vi "FindOutputLine.vi"(8 "error in (no error)":errorcluster, 10 "Line Source":string, 11 "IMAQdx Session In":T1) -> (0 "error out":errorcluster, 2 "Output Line":string, 3 "IMAQdx Session Out":T1)   [LabVIEW 2023]
uses:
  <vilib>/userdefined/High Color/IMAQdx.ctl
  <resource>/objmgr/imaqdx.rc
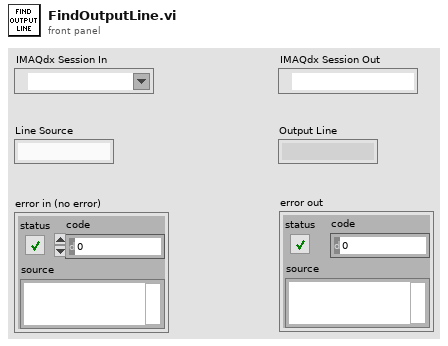
[diagram p1: front panel]
types:
  T1 = typedef "IMAQdx.ctl" = refnum<k21>
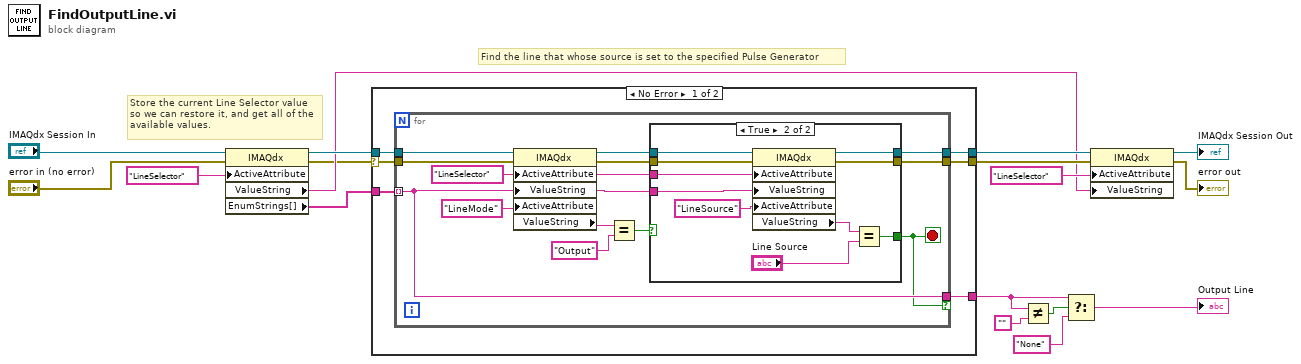
[diagram p0: block diagram]
diagram:
  # "Find the line that whose source is set to the specified Pulse Generator"
  # "Store the current Line Selector value so we can restore it, and get all of the available values."
  n1 = property class="IMAQdx"(reference="IMAQdx Session In", error in="error in (no error)", "ActiveAttribute"="LineSelector") -> (reference out=w16:T1, error out=w1:errorcluster, "ValueString"=w8:string, "EnumStrings[]"=w15:string[])
  n2 = case shown="No Error" w1 {
    selector: w1 -> [w18 w49]
    tunnel: w16 -> [w23 w50]
    tunnel: w15 -> [w22 _]
    tunnel: [w21 w50] -> w11
    tunnel: [w20 w49] -> w9
    tunnel: [w19 _] -> w4
    frame No Error {
      n3 = for {
        tunnel: w23 -> [w36]
        tunnel: w22 -> [w30] mode=indexing
        tunnel: [w30] -> w19 if=w24
        tunnel: [w26] -> w21
        tunnel: w18 -> [w34]
        tunnel: [w25] -> w20
        stop <- w24 stop-if-true
        w31 = "LineSelector" ("ActiveAttribute")
        n4 = property class="IMAQdx"(reference=w36, error in=w34, "ActiveAttribute"=w31, "ValueString"=w30, "ActiveAttribute"="LineMode") -> (reference out=w33:T1, error out=w32:errorcluster, "ValueString"=w29:string)
        n5 = Equal?(x=w29, y="Output" ("ActiveAttribute")) -> (x = y?=w27:bool)
        n6 = case shown="True" w27 {
          tunnel: w33 -> [w38 w48]
          tunnel: w32 -> [w37 w47]
          tunnel: w31 -> [_ w46]
          tunnel: w30 -> [_ w45]
          tunnel: [_ w41] -> w24
          tunnel: [w38 w40] -> w26
          tunnel: [w37 w39] -> w25
          frame False {
          }
          frame True {
            n7 = property class="IMAQdx"(reference=w48, error in=w47, "ActiveAttribute"=w46, "ValueString"=w45, "ActiveAttribute"="LineSource") -> (reference out=w40:T1, error out=w39:errorcluster, "ValueString"=w43:string)
            n8 = Equal?(x=w43, y="Line Source") -> (x = y?=w41:bool)
          }
        }
      }
    }
    frame Error {
    }
  }
  n9 = Not Equal?(x=w4, y="") -> (x != y?=w5:bool)
  n10 = Select(t=w4, s=w5, f="None") -> (s? t:f=→"Output Line":string)
  n11 = property class="IMAQdx"(reference=w11, error in=w9, "ActiveAttribute"="LineSelector", "ValueString"=w8) -> (reference out=→"IMAQdx Session Out":T1, error out=→"error out":errorcluster)
